vi "QBeeper.vi"(8 "error in (no error)":errorcluster, 11 "VISA resource name":refnum<visa-resource-name>) -> (0 "error out":errorcluster, 2 "Beeper State":u32(ring) items=["Off", "On"], 3 "VISA resource name out":refnum<visa-resource-name>)   [LabVIEW 2015, in "Newport 1830-C.lvlib"]
doc: "0=beeper off\n1=beeper on"
uses:
  Newport 1830-C.lvlib
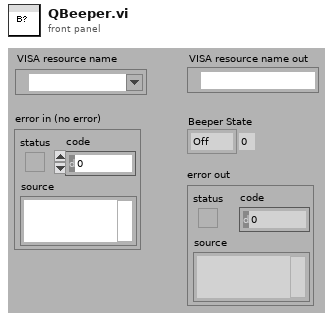
[diagram p1: front panel]
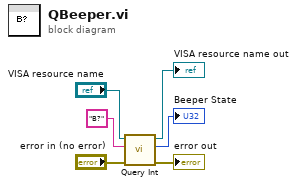
[diagram p0: block diagram]
diagram:
  n1 = call "Query Int.vi"("error in (no error)"="error in (no error)", "write buffer"="B?" ("command"), "VISA resource name In"="VISA resource name") -> ("error out"=→"error out":errorcluster, "int"=→"Beeper State":u32, "VISA resource name out"=→"VISA resource name out":refnum<visa-resource-name>)  [unwired: 6 in]
